vi "Set NICs Enum Ctrl.vi"(8 "Error In":errorcluster, 11 "NIC Info":T1[](array[typedef])) -> (0 "Error Out":errorcluster, 3 "NIC Info":T1[](array[typedef]))   [LabVIEW 2020, in "LMH-LINX.lvlib"]
uses:
  LMH-LINX.lvlib
  NIC Info.ctl
  NIC Mode.ctl
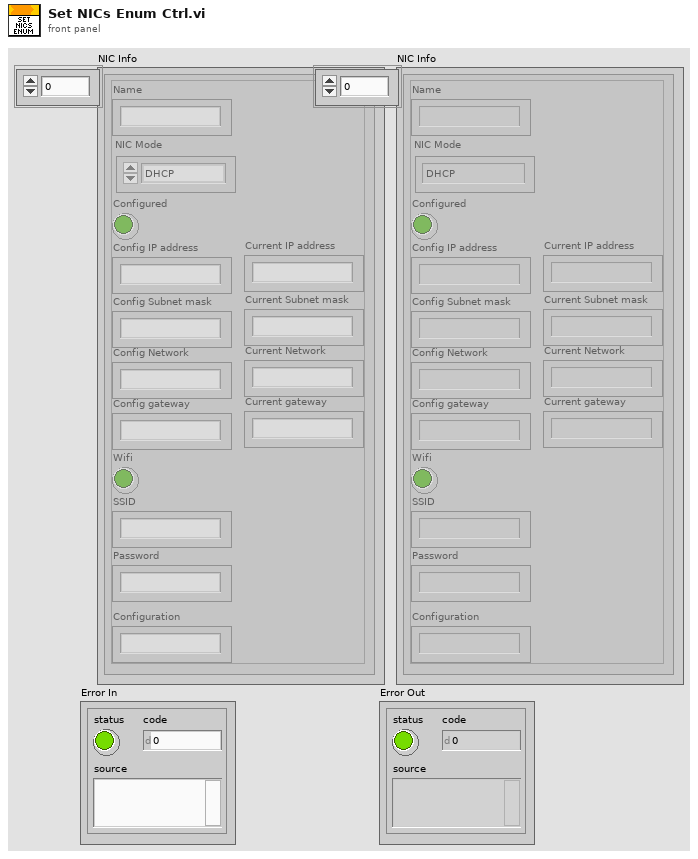
[diagram p1: front panel]
types:
  T1 = typedef "LMH-LINX.lvlib/NIC Info.ctl" = cluster{"Name":string, "NIC Mode":T2, "Configured":bool, "Config IP address":string, "Config Subnet mask":string, "Config Network":string, "Config gateway":string, "Wifi":bool, "SSID":string, "Password":string, "Configuration":string, "Current IP address":string, "Current Subnet mask":string, "Current gateway":string, "Current Network":string}
  T2 = typedef "LMH-LINX.lvlib/NIC Mode.ctl" = enum16{"DHCP", "Static", "Loopback"}
  T3 = typedef "LMH-LINX.lvlib/Network Settings Ctrl Refs.ctl" = cluster{"Hostname":refnum<vi>, "IP address":refnum<vi>, "Subnet mask":refnum<vi>, "Default Gateway":refnum<vi>, "SSID":refnum<vi>, "Password":refnum<vi>, "NIC Status":refnum<vi>, "Network Interface":refnum<vi>, "DCHP":refnum<vi>}
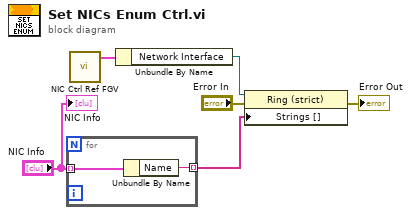
[diagram p0: block diagram]
diagram:
  n1 = for {
    tunnel: "NIC Info" -> [w8] mode=indexing
    tunnel: [w7] -> w1 mode=indexing
    n2 = Unbundle By Name(w8) -> ("Name"=w7:string)
  }
  n3 = call "NIC Ctrl Ref FGV.vi"() -> ("Network Settings Ctrl Refs"=w2:T3)  [unwired: 4 in]
  n4 = Unbundle By Name(w2) -> ("Network Interface"=w4:refnum<vi>)
  n5 = property class="Ring (strict)"(reference=w4, error in="Error In", "Strings []"=w1) -> (error out=→"Error Out":errorcluster)  [unwired: 1 out]
  "NIC Info" <- "NIC Info"
